vi "IGC100 Read Pressure.vi"(4 "error in":errorcluster, 5 "Communication Interval (ms)":u32=1 min=1, 6 "Channel":string="3", 7 "VISA in":refnum<visa-resource-name>="GPIB0::3::INSTR") -> (0 "error out":errorcluster, 2 "Pressure":dbl, 3 "VISA out":refnum<visa-resource-name>)   [LabVIEW 2018]
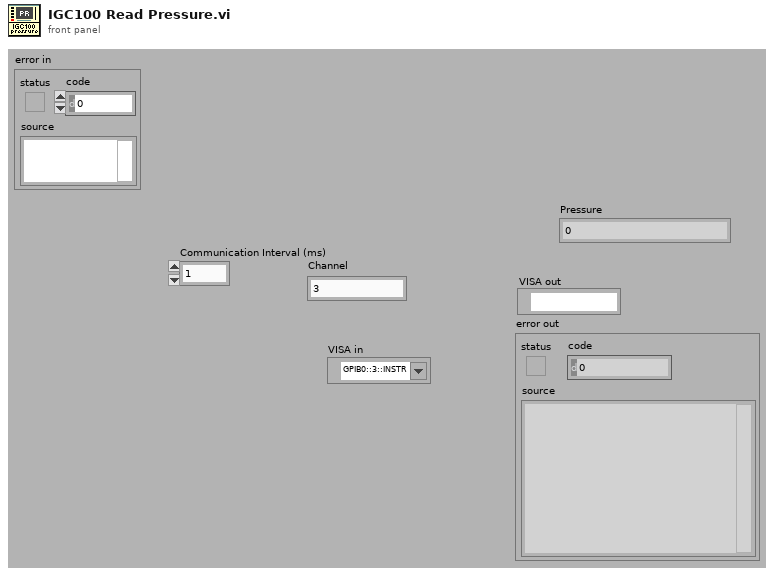
[diagram p1: front panel]
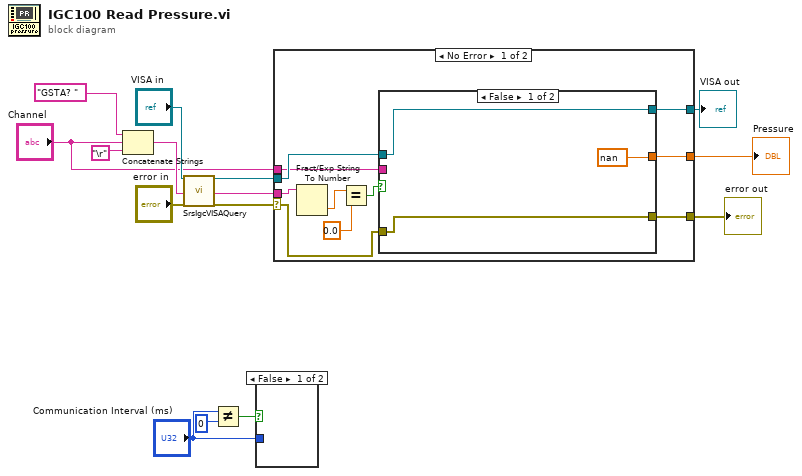
[diagram p0: block diagram]
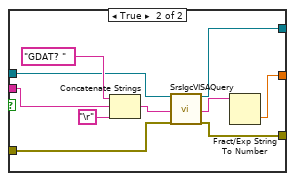
[diagram p2: hidden frame]
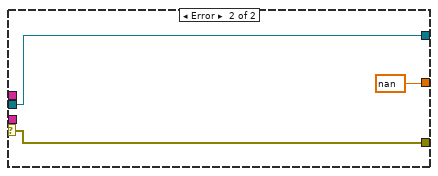
[diagram p3: hidden frame]
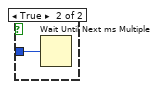
[diagram p4: hidden frame]
diagram:
  n1 = Concatenate Strings("GSTA? ", "Channel", "\r") -> (w15:string)
  n2 = call "SrsIgcVISAQuery.vi"("VISA in"="VISA in", "Command"=w15, "error in"="error in") -> ("VISA out"=w6:refnum<visa-resource-name>, "Output"=w5:string, "error out"=w7:errorcluster)  [unwired: 14 in]
  n3 = Not Equal?(x="Communication Interval (ms)", y=u32 0) -> (x != y?=w10:bool)
  n4 = case shown="False" w10 {
    tunnel: "Communication Interval (ms)" -> [_ w16]
    frame False {
    }
    frame True {
      n5 = Wait Until Next ms Multiple(millisecond multiple=w16) -> ()  [unwired: 1 out]
    }
  }
  n6 = case shown="No Error" w7 {
    selector: w7 -> [w22 w41]
    tunnel: w6 -> [w21 w42]
    tunnel: w5 -> [w25 _]
    tunnel: "Channel" -> [w20 _]
    tunnel: [w19 nan] -> w3
    tunnel: [w18 w41] -> w2
    tunnel: [w17 w42] -> w1
    frame No Error {
      n7 = Fract/Exp String To Number(string=w25) -> (number=w24:dbl)  [unwired: 3 in, 1 out]
      n8 = Equal?(x=w24, y=0.0) -> (x = y?=w26:bool)
      n9 = case shown="False" w26 {
        tunnel: w22 -> [w28 w34]
        tunnel: w21 -> [w29 w35]
        tunnel: w20 -> [_ w37]
        tunnel: [nan w33] -> w19
        tunnel: [w28 w31] -> w18
        tunnel: [w29 w30] -> w17
        frame False {
        }
        frame True {
          n10 = Concatenate Strings("GDAT? ", w37, "\r") -> (w36:string)
          n11 = call "SrsIgcVISAQuery.vi"("VISA in"=w35, "Command"=w36, "error in"=w34) -> ("VISA out"=w30:refnum<visa-resource-name>, "Output"=w32:string, "error out"=w31:errorcluster)  [unwired: 14 in]
          n12 = Fract/Exp String To Number(string=w32) -> (number=w33:dbl)  [unwired: 3 in, 1 out]
        }
      }
    }
    frame Error {
    }
  }
  "Pressure" <- w3
  "VISA out" <- w1
  "error out" <- w2
